vi "SEA-9811_ReceiverAndTransmitter_FPGA.vi"() -> ()   [LabVIEW 2012]
doc: "This example demonstrates the receiver's functionality. ARINC data can be received with up to 8 channels which can be configured regarding high- or low-speed data rate, label recognition, parity check, decoder functions or label bit order (CONFIG). Up to sixteen 8-bit labels can be stored for label recognition. Duplicate values if you need fewer labels. For more details, look at the RT frontend example.\n\nCopyright (c) 2013 S.E.A. Datentechnik GmbH, Germany"
uses:
  <vilib>/Platform/TimedLoop/XDataNode/timing_clust.ctl
  <vilib>/Platform/TimedLoop/XDataNode/nitl_modes.ctl
  <vilib>/Platform/TimedLoop/XDataNode/wakeup.ctl
  <vilib>/rvi/eio/common/nirviEmuTemplateMethod_errors.vi
  <vilib>/rvi/Emulation/niFpgaSctlEmulationGetInTimedLoop.vi
  <vilib>/rvi/Emulation/niFpgaSctlEmulationGlobalWrite.vi
  <vilib>/rvi/eio/common/nirviEmuTemplatePropertyGet_noerrors.vi
  <vilib>/rvi/interface/RandomDataEmulation/nirviRandomDataFPGAFIFO.vi
  <vilib>/rvi/interface/RandomDataEmulation/niFpgaRandomDataHandleErrors.vi
  <vilib>/rvi/Emulation/niFpgaSctlEmulationRegisterWithScheduler.vi
  <vilib>/rvi/Emulation/niFpgaSctlEmulationScheduler.vi
  <vilib>/Platform/TimedLoop/XDataNode/XDataNode.xnode
  <vilib>/eio/EIOMethodNode/EIOMethodNode.xnode
  <vilib>/eio/EIONode/EIONode.xnode
  <vilib>/eio/EIOPropertyNode/EIOPropertyNode.xnode
  <vilib>/rvi/DataTransferAndStorage/Container/XNode/niFpgaContainer.xnode
  <vilib>/rvi/interface/RandomDataEmulation/nirviRandomDataFpgaReadWriteTemplate.vi
  <vilib>/rvi/eio/common/nirviEmuTemplatePropertyGet_errors.vi
  <vilib>/rvi/eio/common/nirviEmuTemplatePropertySet_errors.vi
  <vilib>/rvi/eio/common/nirviEmuTemplatePropertySet_noerrors.vi
  <userlib>/FPGA Timekeeper 1.1b0/FPGA Timekeeper.lvlib
  <vilib>/Platform/TimedLoop/XDataNode/XDNodeRunTimeDep.lvlib
panel:
  in  "Rx Label Filter":u8[](array[numeric])=[0, 0, 0, 0, 0, 0, 0, 0, 0, 0, 0, 0, 0, 0, 0, 0]
  out "Rx rate us":u32
  out "Elements in FIFO":u32
  out "FPGA Timekeeper time (ns)":u64
  out "FPGA Timekeeper locked":bool
  out "offset from RT time (ns)":i32
  in  "RT time (ns)":u64
  in  "Finished config":bool
  in  "Configure\nchannel":bool
  out "Rx Status":u16 format="%016b"
  out "Tx Status":u8 format="%08b"
  in  "Tx Data":u32=305419896 format="%08x"
  in  "Tx Config Data (TCR)":u16=8192 format="%04x"
  in  "Transmit Data":bool
  out "DMA Overflow":bool
  in  "Rx Channel Number":u8 max=7 step=1
  in  "Rx Config Data (RCR)":u16=32 format="%04x"
  # "Please refer to VI description for instructions!"
  # "Receiver Configuration"
  # "DMA Status"
  # "Transmitter"
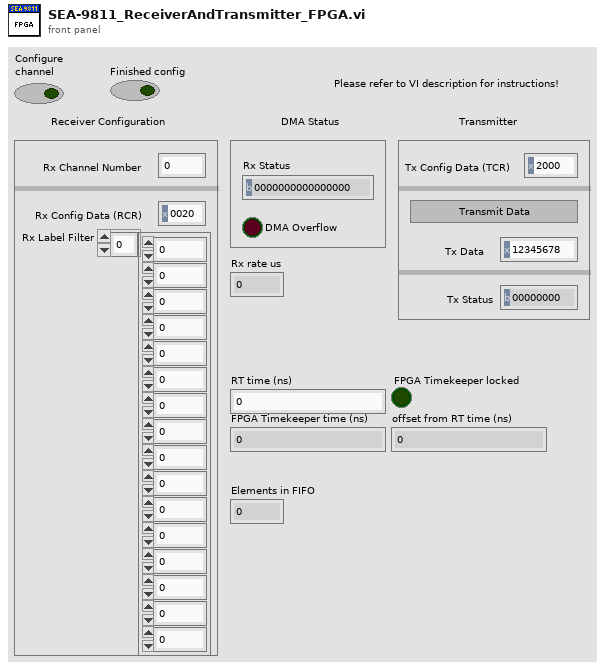
[diagram p1: front panel]
types:
  T1 = cluster{"Rx Label Filter[0]":u8, "Rx Label Filter[1]":u8, "Rx Label Filter[2]":u8, "Rx Label Filter[3]":u8, "Rx Label Filter[4]":u8, "Rx Label Filter[5]":u8, "Rx Label Filter[6]":u8, "Rx Label Filter[7]":u8, "Rx Label Filter[8]":u8, "Rx Label Filter[9]":u8, "Rx Label Filter[10]":u8, "Rx Label Filter[11]":u8, "Rx Label Filter[12]":u8, "Rx Label Filter[13]":u8, "Rx Label Filter[14]":u8, "Rx Label Filter[15]":u8}
  T2 = typedef "XDNodeRunTimeDep.lvlib/timing_clust.ctl" = cluster{"Expected End [f-1]":u64, "Actual End [f-1]":u64, "Finished Late? [f-1]":bool, "Expected End [i-1]":u64, "Actual End [i-1]":u64, "Finished Late? [i-1]":bool, "Expected Start [i]":u64, "Actual Start [i]":u64, "Expected Start [f]":u64, "Actual Start [f]":u64, "Source Name":string, "Structure Name":string, "Period":i64, "Deadline":i64, "Offset":i64, "Start":i64, "Priority":i32, "Timeout":i32, "Mode":T3, "Wakeup Reason":T4, "Error":errorcluster, "Source Type":string, "Secondary Source Type":string, "Global End Time":u64, "Global Start Time":u64, "Frame Duration":u64, "Iteration Duration":u64, "Assigned CPU":i32, "I/O Scan Engine Mode":u32}
  T3 = typedef "XDNodeRunTimeDep.lvlib/nitl_modes.ctl" = enum32{"No Change", "Process missed periods, maintain original phase", "Discard missed periods, maintain original phase", "Process missed periods, ignore original phase", "Discard missed periods, ignore original phase"}
  T4 = typedef "XDNodeRunTimeDep.lvlib/wakeup.ctl" = enum32{"Normal", "Aborted", "Asynchronous wakeup", "Timing source error", "Timed loop error", "Timeout"}
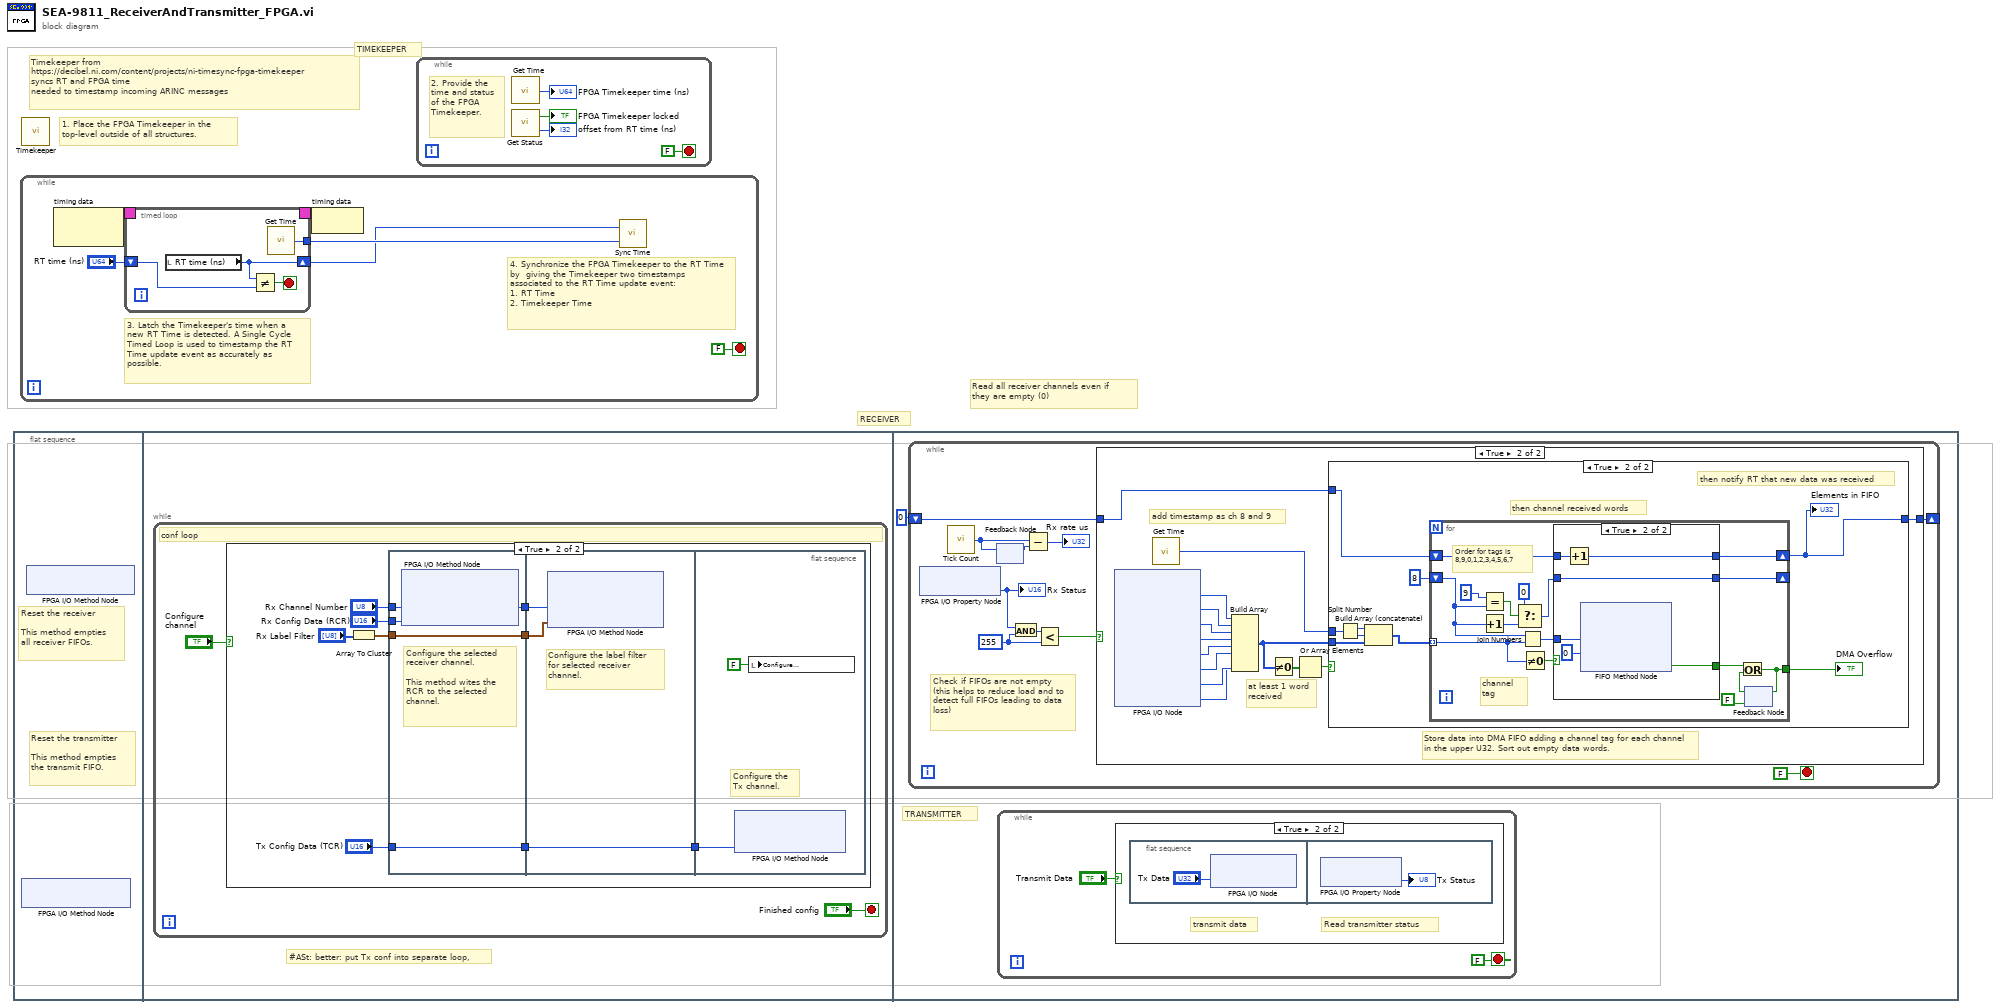
[diagram p0: block diagram]
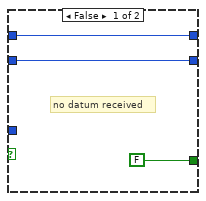
[diagram p6: hidden frame]
diagram:
  # "Read all receiver channels even if they are empty (0)"
  # "TIMEKEEPER"
  # "Timekeeper from\nhttps://decibel.ni.com/content/projects/ni-timesync-fpga-timekeeper\nsyncs RT and FPGA time\nneeded to timestamp incoming ARINC messages"
  # "1. Place the FPGA Timekeeper in the top-level outside of all structures."
  # "RECEIVER"
  n1 = flat-sequence {
    frame #0 {
      # "Reset the transmitter\n\nThis method empties\nthe transmit FIFO."
      # "Reset the receiver\n\nThis method empties\nall receiver FIFOs."
      n2 = xnode "FPGA I/O Method Node"() -> ()  [unwired: 1 in, 1 out]
      n3 = xnode "FPGA I/O Method Node"() -> ()  [unwired: 1 in, 1 out]
    }
    frame #1 {
      # "#ASt: better: put Tx conf into separate loop,"
      n4 = while {
        stop <- "Finished config" stop-if-true
        # "conf loop"
        n5 = case shown="True" "Configure\nchannel" {
          frame False {
          }
          frame True {
            n6 = Array To Cluster(array="Rx Label Filter") -> (cluster=w3:T1)
            n7 = flat-sequence {
              tunnel: "Rx Channel Number" -> [w15]
              tunnel: [w15] -> w11
              tunnel: "Rx Config Data (RCR)" -> [w14]
              tunnel: [w13] -> w10
              tunnel: w3 -> [w13]
              tunnel: "Tx Config Data (TCR)" -> [w12]
              tunnel: [w12] -> w5
              tunnel: w11 -> [w18]
              tunnel: w10 -> [w17]
              tunnel: [w16] -> w6
              tunnel: w5 -> [w16]
              tunnel: w6 -> [w20]
              frame #0 {
                # "Configure the selected\nreceiver channel.\n\nThis method wites the\nRCR to the selected\nchannel."
                n8 = xnode "FPGA I/O Method Node"("Channel Number"=w15, "Control Register"=w14) -> ()  [unwired: 1 in, 1 out]
              }
              frame #1 {
                # "Configure the label filter\nfor selected receiver\nchannel."
                n9 = xnode "FPGA I/O Method Node"("Channel Number"=w18, "Label Filter"=w17) -> ()  [unwired: 1 in, 1 out]
              }
              frame #2 {
                # "Configure the\nTx channel."
                n10 = xnode "FPGA I/O Method Node"("Control Register"=w20) -> ()  [unwired: 1 in, 1 out]
                n11 = local write "Configure\nchannel"(FALSE ("Configure\nchannel")) -> ()
              }
            }
          }
        }
      }
    }
    frame #2 {
      # "TRANSMITTER"
      n12 = while {
        shift-right: [w29] -> _
        shift-left: u32 0 -> [w30]
        stop <- FALSE stop-if-true
        w32 = u16 255 ("y")
        # "Check if FIFOs are not empty\n(this helps to reduce load and to detect full FIFOs leading to data loss)"
        n13 = xnode "FPGA I/O Property Node"() -> ("Rx Status"=w34:u16)  [unwired: 1 in, 1 out]
        "Rx Status" <- w34
        n14 = call "Tick Count"() -> ("Tick Count(uSec)"=w28:u32)
        n15 = feedback-in #1(w28) -> ()
        n16 = feedback #1() -> (w27:u32)  [unwired: 1 in]
        n17 = And(x=w34, y=w32) -> (x .and. y?=w33:u16)
        n18 = Subtract(x=w28, y=w27) -> (x-y=→"Rx rate us":u32)
        n19 = Less?(x=w33, y=w32) -> (x < y?=w31:bool)
        n20 = case shown="True" w31 {
          tunnel: w30 -> [w36 w42]
          tunnel: [w36 w41] -> w29
          frame False {
          }
          frame True {
            # "add timestamp as ch 8 and 9"
            # "at least 1 word\nreceived"
            # "Store data into DMA FIFO adding a channel tag for each channel in the upper U32. Sort out empty data words."
            n21 = xnode "FPGA I/O Node"() -> ("Mod1/Rx0"=w44:u32, "Mod1/Rx1"=w45:u32, "Mod1/Rx2"=w46:u32, "Mod1/Rx3"=w47:u32, "Mod1/Rx4"=w48:u32, "Mod1/Rx5"=w49:u32, "Mod1/Rx6"=w50:u32, "Mod1/Rx7"=w43:u32)  [unwired: 8 in, 8 out]
            n22 = call <userlib>:"Get Time.vi"() -> ("time (ns)"=w37:u64)
            n23 = Build Array(w44, w45, w46, w47, w48, w49, w50, w43) -> (w40:u32[])
            n24 = Not Equal To 0?(x=w40) -> (x != 0?=w39:bool[])
            n25 = Or Array Elements(Boolean array=w39) -> (logical OR=w38:bool)
            n26 = case shown="True" w38 {
              tunnel: w42 -> [w51 w52]
              tunnel: [w51 w60] -> w41
              tunnel: w40 -> [_ w57]
              tunnel: w37 -> [_ w53]
              frame False {
              }
              frame True {
                # "then notify RT that new data was received"
                # "then channel received words"
                n27 = Split Number(x=w53) -> (hi(x)=w55:u32, lo(x)=w54:u32)
                n28 = Build Array (concatenate)(w55, w54, w57) -> (w56:u32[])
                n29 = for {
                  tunnel: w56 -> [w68] mode=indexing
                  tunnel: [w73] -> w59
                  shift-right: [w69] -> w60
                  shift-left: w52 -> [w70]
                  shift-right: [w61] -> _
                  shift-left: u32 8 ("hi") -> [w65]
                  # "Order for tags is\n8,9,0,1,2,3,4,5,6,7"
                  # "channel\ntag"
                  n30 = Equal?(x=u32 9, y=w65) -> (x = y?=w66:bool)
                  n31 = Increment(x=w65) -> (x+1=w67:u32)
                  n32 = Select(t=u32 0, s=w66, f=w67) -> (s? t:f=w62:u32)
                  n33 = Join Numbers(hi=w65, lo=w68) -> ((hi.lo)=w71:u64)
                  n34 = Not Equal To 0?(x=w68) -> (x != 0?=w72:bool)
                  n35 = case shown="True" w72 {
                    tunnel: [FALSE ("Timed Out?") w85] -> w74
                    tunnel: w71 -> [_ w82]
                    tunnel: w70 -> [w78 w84]
                    tunnel: [w78 w83] -> w69
                    tunnel: w62 -> [w77 w80]
                    tunnel: [w77 w80] -> w61
                    frame False {
                      # "no datum received"
                    }
                    frame True {
                      n36 = Increment(x=w84) -> (x+1=w83:u32)
                      n37 = xnode ("FIFO Method Node")("Element"=w82, "Timeout"=0) -> ("Timed Out?"=w85:bool)  [unwired: 1 in, 1 out]
                    }
                  }
                  n38 = feedback #2(FALSE) -> (w75:bool)
                  n39 = Or(x=w74, y=w75) -> (x .or. y?=w73:bool)
                  n40 = feedback-in #2(w73) -> ()
                }
                "DMA Overflow" <- w59
                "Elements in FIFO" <- w60
              }
            }
          }
        }
      }
      n41 = while {
        stop <- FALSE stop-if-true
        n42 = case shown="True" "Transmit Data" {
          frame False {
          }
          frame True {
            # "Read transmitter status"
            # "transmit data"
            n43 = flat-sequence {
              frame #0 {
                n44 = xnode "FPGA I/O Node"("Mod1/Tx0"="Tx Data") -> ()  [unwired: 1 in, 1 out]
              }
              frame #1 {
                n45 = xnode "FPGA I/O Property Node"() -> ("Tx Status"=→"Tx Status":u8)  [unwired: 1 in, 1 out]
              }
            }
          }
        }
      }
    }
  }
  n46 = while {
    stop <- FALSE stop-if-true
    # "3. Latch the Timekeeper's time when a new RT Time is detected. A Single Cycle Timed Loop is used to timestamp the RT Time update event as accurately as possible."
    # "4. Synchronize the FPGA Timekeeper to the RT Time by  giving the Timekeeper two timestamps associated to the RT Time update event:\n1. RT Time\n2. Timekeeper Time"
    n47 = node-c288() -> (w91:T2)  [unwired: 1 in]
    n48 = timed-loop {
      timing: w91 -> [_]
      timing-out: [_] -> w90
      shift-right: [w92] -> w86
      shift-left: "RT time (ns)" -> [w93]
      tunnel: [w95] -> w89
      stop <- w94 stop-if-true
      n49 = local read "RT time (ns)"() -> (w92:u64)
      n50 = Not Equal?(x=w92, y=w93) -> (x != y?=w94:bool)
      n51 = call <userlib>:"Get Time.vi"() -> ("time (ns)"=w95:u64)
    }
    n52 = node-c288(w90) -> ()
    n53 = call <userlib>:"Sync Time.vi"("FPGA Timekeeper time (ns)"=w89, "time reference time (ns)"=w86) -> ()
  }
  n54 = call <userlib>:"Timekeeper.vi"() -> ()  [unwired: 12 in]
  n55 = while {
    stop <- FALSE stop-if-true
    # "2. Provide the time and status of the FPGA Timekeeper."
    n56 = call <userlib>:"Get Time.vi"() -> ("time (ns)"=→"FPGA Timekeeper time (ns)":u64)
    n57 = call <userlib>:"Get Status.vi"() -> ("FPGA Timekeeper locked"=→"FPGA Timekeeper locked":bool, "offset from time reference"=→"offset from RT time (ns)":i32)
  }
